vi "Get VI Library.vi"(11 "VI Refnum":refnum<vi>) -> (1 "Library":refnum<vi>, 2 "VI thinks it is owned by a library":bool)   [LabVIEW 2021]
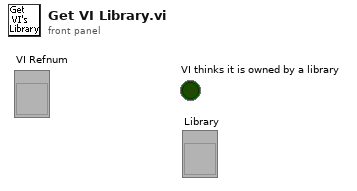
[diagram p1: front panel]
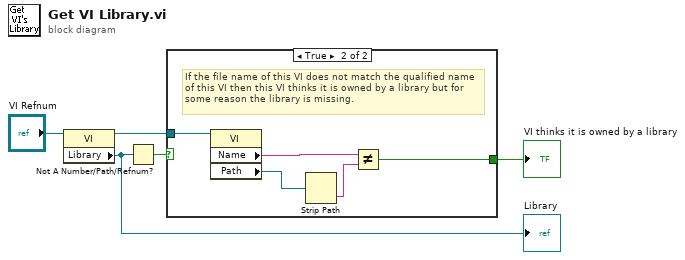
[diagram p0: block diagram]
diagram:
  n1 = property class="VI"(reference="VI Refnum") -> (reference out=w3:refnum<vi>, "Library"=w1:refnum<vi>)  [unwired: 1 in, 1 out]
  "Library" <- w1
  n2 = Not A Number/Path/Refnum?(number/path/refnum=w1) -> (NaN/Path/Refnum?=w4:bool)
  n3 = case shown="True" w4 {
    tunnel: w3 -> [_ w9]
    tunnel: [_ w6] -> w2
    frame False {
    }
    frame True {
      # "If the file name of this VI does not match the qualified name of this VI then this VI thinks it is owned by a library but for some reason the library is missing."
      n4 = property class="VI"(reference=w9) -> ("Name"=w7:string, "Path"=w8:path)  [unwired: 1 in, 2 out]
      n5 = Strip Path(path=w8) -> (name=w10:string)  [unwired: 1 out]
      n6 = Not Equal?(x=w7, y=w10) -> (x != y?=w6:bool)
    }
  }
  "VI thinks it is owned by a library" <- w2
